vi "Generator Lesson 1.vi"() -> ()   [LabVIEW 2019]
uses:
  <vilib>/Instr/_visa.llb/VISA Configure Serial Port (Instr).vi
panel:
  in  "generator":refnum<visa-resource-name>
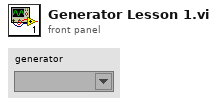
[diagram p1: front panel]
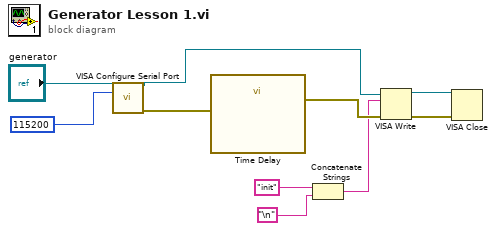
[diagram p0: block diagram]
diagram:
  n1 = call-poly "VISA Configure Serial Port"("VISA resource name"="generator", "baud rate (9600)"=u32 115200) -> ("VISA resource name out"=w7:refnum<visa-resource-name>, "error out"=w8:errorcluster)  [unwired: 12 in]
  n2 = call "Time Delay"("error in (no error)"=w8) -> ("error out"=w6:errorcluster)  [unwired: 10 in]
  n3 = Concatenate Strings("init", "\n") -> (w3:string)
  n4 = VISA Write(VISA resource name=w7, write buffer=w3, error in (no error)=w6) -> (VISA resource name out=w2:refnum<visa-resource-name>, error out=w1:errorcluster)  [unwired: 1 out]
  n5 = VISA Close(VISA resource name=w2, error in (no error)=w1) -> ()  [unwired: 1 out]
